vi "set_gate_parameters.vi"(4 "repetitions":i64, 5 "pulse duration (iterations)":i64, 6 "offset duration (iterations)":i64, 7 "clock index":i32, 8 "error in (no error)":errorcluster, 9 "low phase duration (iterations)":i64, 10 "high phase duration (iterations)":i64, 11 "FPGAWrapperMH120124FrameScan_PXI7813R in":refnum<class "FPGAWrapperMH120124FrameScan_PXI7813R.lvclass">) -> (0 "error out":errorcluster, 3 "FPGAWrapperMH120124FrameScan_PXI7813R out":refnum<class "FPGAWrapperMH120124FrameScan_PXI7813R.lvclass">)   [LabVIEW 2010, in "FPGAWrapperMH120124FrameScan_PXI7813R.lvclass"]
uses:
  FPGAWrapperMH120124FrameScan_PXI7813R.lvclass
  common_typedefs/gate_parameters_cluster.ctl
  fpgaVIsAndControls/gate_cluster.ctl
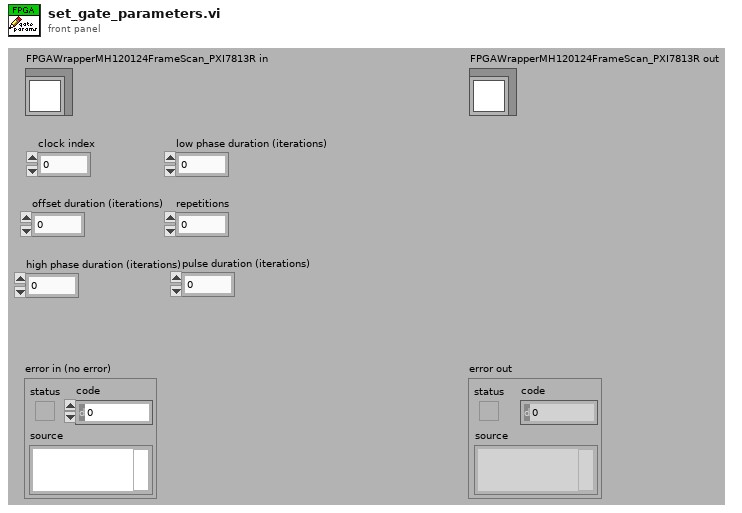
[diagram p1: front panel]
types:
  T1 = typedef "gate_cluster.ctl" = cluster{"index":i32, "parameters":T2}
  T2 = typedef "gate_parameters_cluster.ctl" = cluster{"offset":i64, "pulsing":i64, "not pulsing":i64, "cycles per pulse":i64, "repetitions":i64}
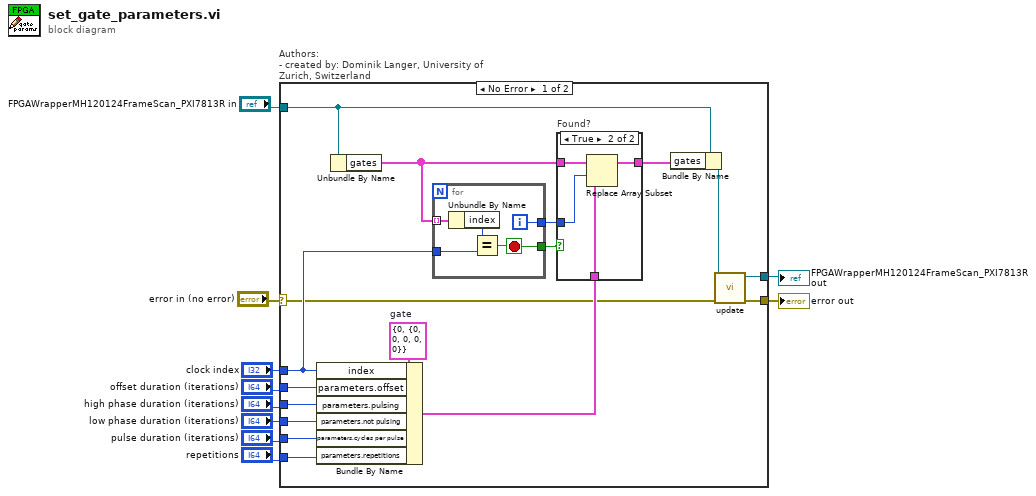
[diagram p0: block diagram]
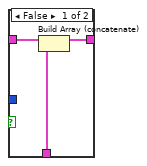
[diagram p2: hidden frame]
diagram:
  n1 = case "Authors: \n- created by: Dominik Langer, University of Zurich, Switzerland" shown="No Error" "error in (no error)" {
    selector: "error in (no error)" -> [w12 w40]
    tunnel: "FPGAWrapperMH120124FrameScan_PXI7813R in" -> [w22 w41]
    tunnel: [w13 w41] -> w10
    tunnel: [w11 w40] -> w9
    tunnel: "clock index" -> [w21 _]
    tunnel: "repetitions" -> [w27 _]
    tunnel: "high phase duration (iterations)" -> [w26 _]
    tunnel: "offset duration (iterations)" -> [w25 _]
    tunnel: "low phase duration (iterations)" -> [w24 _]
    tunnel: "pulse duration (iterations)" -> [w23 _]
    frame No Error {
      w15 = T1 {"index"=0, "parameters"={"offset"=0, "pulsing"=0, "not pulsing"=0, "cycles per pulse"=0, "repetitions"=0}}  # gate
      n2 = Bundle By Name(cluster=w15, "index"=w21, "parameters.offset"=w25, "parameters.pulsing"=w26, "parameters.not pulsing"=w24, "parameters.cycles per pulse"=w23, "parameters.repetitions"=w27) -> (w17:T1)
      n3 = Unbundle By Name(w22) -> ("gates"=w20:T1[])
      n4 = for {
        tunnel: w20 -> [w39] mode=indexing
        tunnel: w21 -> [w38]
        tunnel: [w36] -> w18
        tunnel: [w35] -> w16
        i -> [w36]
        stop <- w35 stop-if-true
        n5 = Unbundle By Name(w39) -> ("index"=w37:i32)
        n6 = Equal?(x=w37, y=w38) -> (x = y?=w35:bool)
      }
      n7 = case "Found?" shown="True" w16 {
        tunnel: w20 -> [w30 w34]
        tunnel: [w28 w33] -> w19
        tunnel: w18 -> [_ w32]
        tunnel: w17 -> [w29 w31]
        frame False {
          n8 = Build Array (concatenate)(w30, w29) -> (w28:T1[])
        }
        frame True {
          n9 = Replace Array Subset(array=w34, new element=w31, index=w32) -> (w33:T1[])
        }
      }
      n10 = Bundle By Name(cluster=w22, "gates"=w19) -> (w14:refnum<class "FPGAWrapperMH120124FrameScan_PXI7813R.lvclass">)
      n11 = call-dynamic "update.vi"("error in (no error)"=w12, "FPGAWrapperMH120124FrameScan_PXI7813R in"=w14) -> ("error out"=w11:errorcluster, "FPGAWrapperMH120124FrameScan_PXI7813R out"=w13:refnum<class "FPGAWrapperMH120124FrameScan_PXI7813R.lvclass">)  [unwired: 8 in]
    }
    frame Error {
    }
  }
  "error out" <- w9
  "FPGAWrapperMH120124FrameScan_PXI7813R out" <- w10
